vi "Change password GUI.vi"(6 "User access cluster in":T1 {"Expire sec" format="%.2f"}, 8 "error in (no error)":errorcluster, 10 "New user?":bool, 11 "Filepath":path=path "C:/Documents and Settings/default/Desktop/New Folder/passwords.log") -> (0 "error out":errorcluster, 1 "Activity log out":T3 {"Epoch sec" format="%.2e"}, 2 "Cancelled?":bool, 4 "User access cluster out":T1 {"Expire sec" format="%.2f"})   [LabVIEW 2013]
doc: "This is a pop-up panel which lets the user to enter a new password or click cancel (if \"New user?\" = F). It is a modal GUI.\n\nIt uses a filepath to an encrypted password file. If there is a file read error a custom error code is returned (error not announced here). \n\nIf called with \"New user?\" = F the user must enter both old and new passwords, else the old password is filled automaticallly from the \"User access cluster in\". The prompt also changes depending on the state of the \"new user?\" input.\n\nWhen the user clicks OK, the code:\n1) checks that old password is valid for this user, if not, it is announced, and this vi returns.\n2) checks that the two new passwords are identical. If not, user is informed and the vi waits for another continue or cancel (if enabled).\n3) If the two new passwords are equal, they are checked for minimum length of \"Min password char\" (from access configuration cluster) characters. If not of sufficient length, user is informed, and this vi waits for continue or cancel.\n4) finally, if new passwords are equal and valid this vi writes the new password to file. Also, if the user was a new user, this field is set to false in the password file.\n\n If the user changes the pasword it is recorded in the activity log, which can be written to an activity log file by subsequent vis."
uses:
  User Access Type defs/Acitivity cluster array.ctl
  User Access Type defs/Acitivity cluster.ctl
  User Access Type defs/User access cluster.ctl
  User Access Type defs/Security level U8.ctl
panel:
  in  "New password 2":string caption="New password\n(repeat)"
  in  "New password":string
  out "State case":string
  in  "Old password":string
  in  "Boolean 2":bool
  in  "Boolean":bool
  out "prompt":string="Enter your old password and the new password (twice)"
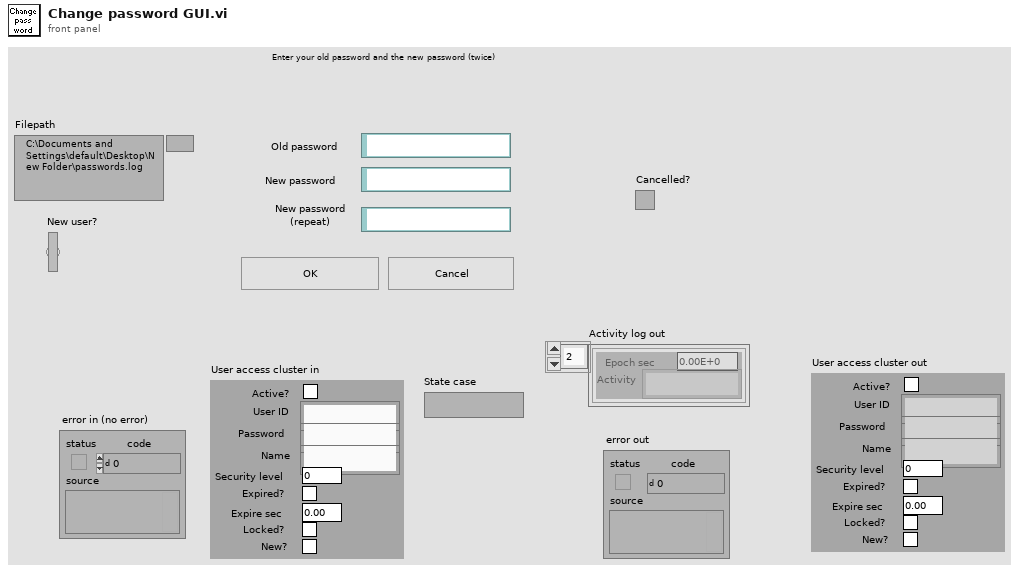
[diagram p1: front panel]
types:
  T1 = typedef "User access cluster.ctl" = cluster{"Active?":bool, "User ID":string, "Password":string, "Name":string, "Security level":T2, "Expired?":bool, "Expire sec":dbl, "Locked?":bool, "New?":bool}
  T2 = typedef "Security level U8.ctl" = u8
  T3 = typedef "Acitivity cluster array.ctl" = T4[]
  T4 = typedef "Acitivity cluster.ctl" = cluster{"Epoch sec":dbl, "Activity":string}
  T5 = typedef "All users access configuration cluster.ctl" = cluster{"Max ID attempts":i32, "Max password attempts":i32, "Expiration enabled":bool, "Expire days":i32, "User array":T6, "Min password char":i32}
  T6 = typedef "User access cluster array.ctl" = T1[]
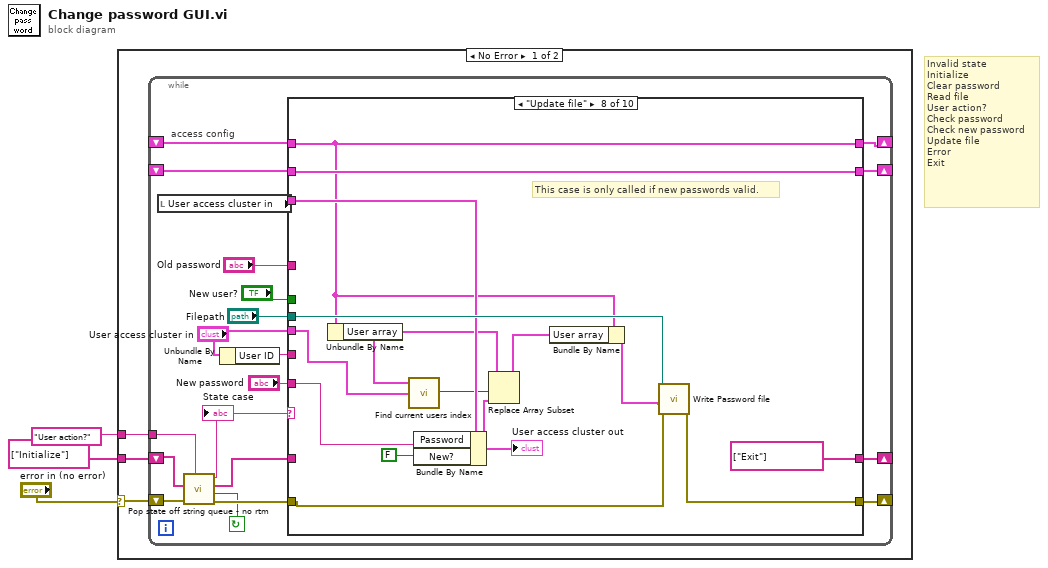
[diagram p0: block diagram]
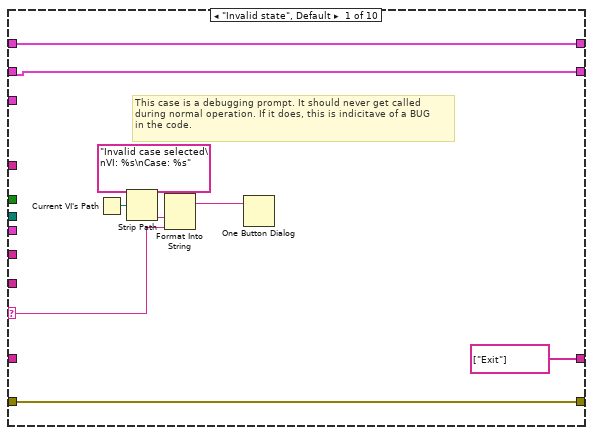
[diagram p2: hidden frame]
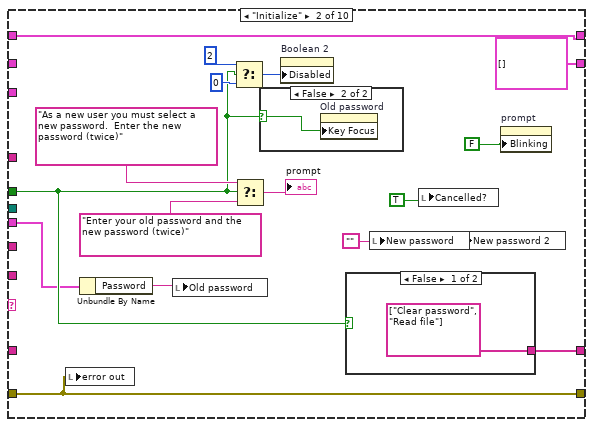
[diagram p3: hidden frame]
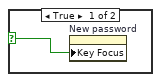
[diagram p4: hidden frame]
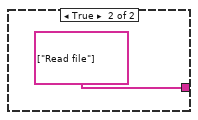
[diagram p5: hidden frame]
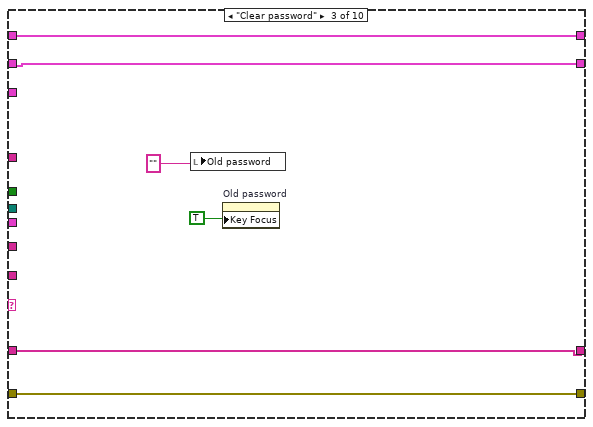
[diagram p6: hidden frame]
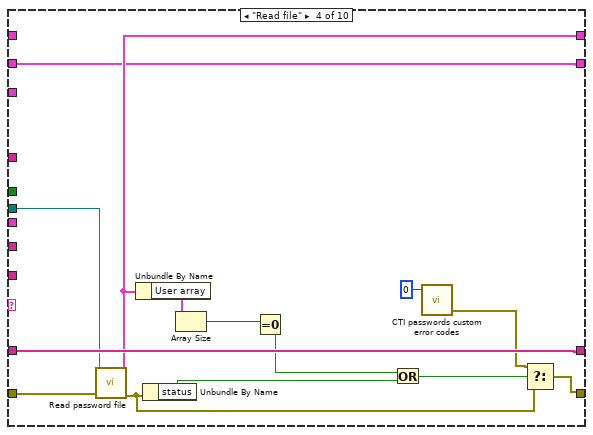
[diagram p7: hidden frame]
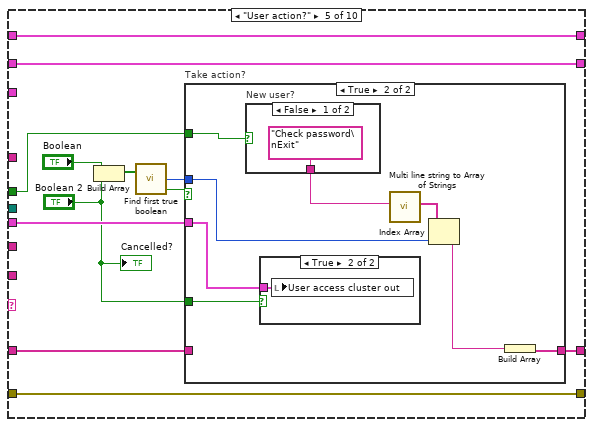
[diagram p8: hidden frame]
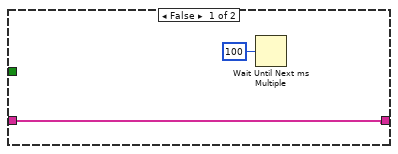
[diagram p9: hidden frame]
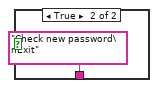
[diagram p11: hidden frame]
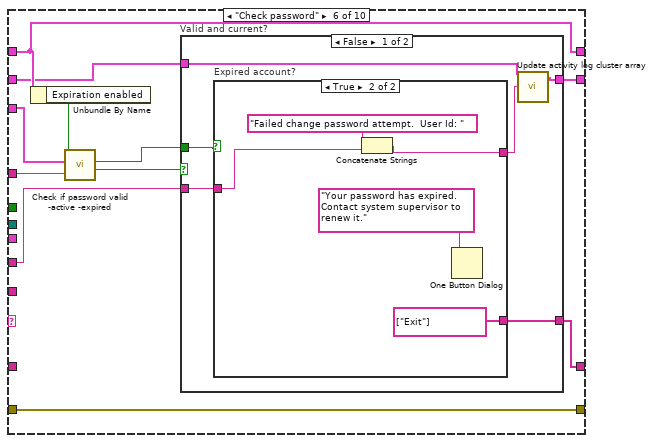
[diagram p12: hidden frame]
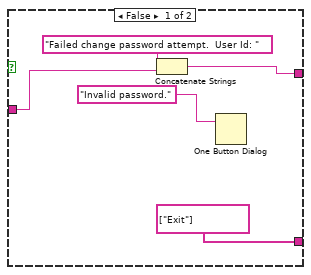
[diagram p13: hidden frame]
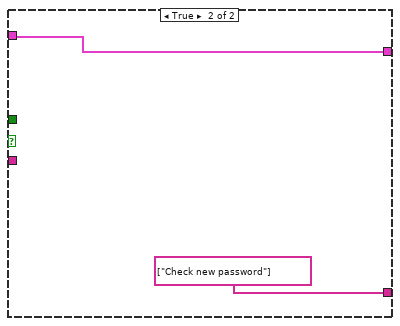
[diagram p14: hidden frame]
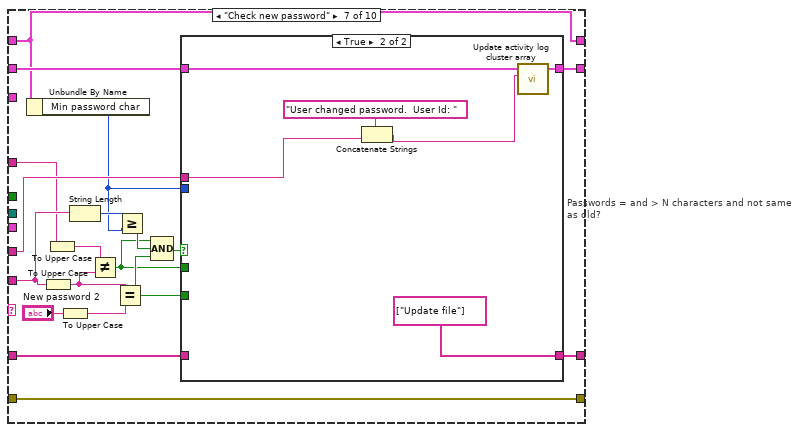
[diagram p15: hidden frame]
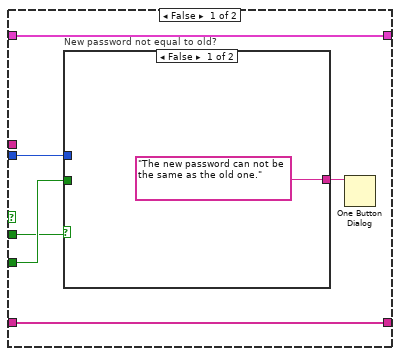
[diagram p16: hidden frame]
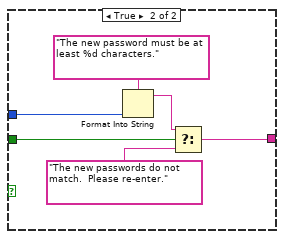
[diagram p17: hidden frame]
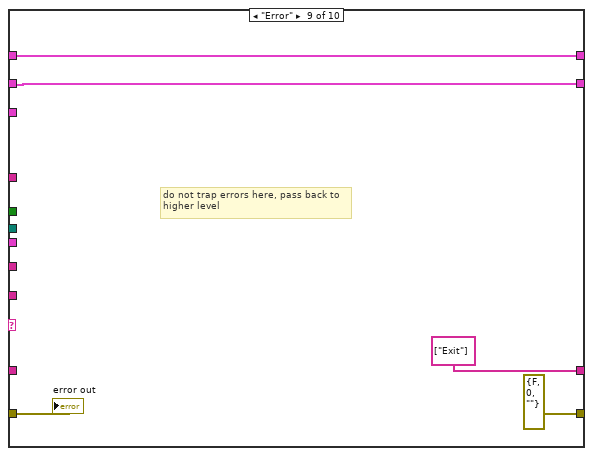
[diagram p18: hidden frame]
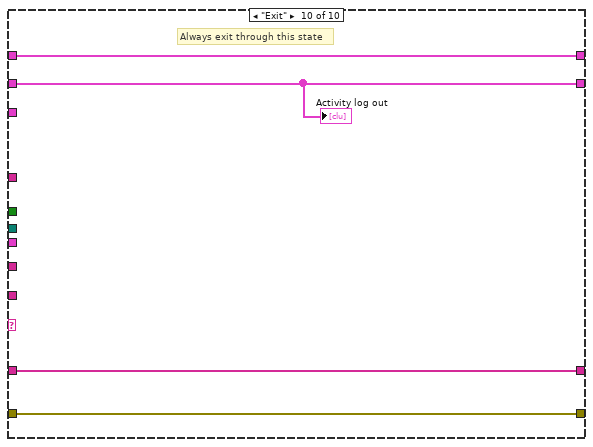
[diagram p19: hidden frame]
diagram:
  # "Invalid state\nInitialize\nClear password\nRead file\nUser action?\nCheck password\nCheck new password\nUpdate file\nError\nExit"
  n1 = case shown="No Error" "error in (no error)" {
    selector: "error in (no error)" -> [w6 _]
    tunnel: string[] ["Initialize"] ("State que out") -> [w5 _]
    tunnel: "User action?" ("Default state") -> [w4 _]
    frame No Error {
      n2 = while {
        tunnel: w4 -> [w18]
        shift-left: w5 -> [w22]
        shift-right: [w20] -> _
        shift-left: w6 -> [w26]
        shift-right: [w24] -> _
        shift-right: [w16] -> _
        shift-left: _ -> [w17]
        shift-right: [w15] -> _
        shift-left: _ -> [w14]
        stop <- w19 continue-if-true
        # "access config"
        n3 = local read "User access cluster in"() -> (w12:T1)
        n4 = call "Pop state off string queue - no rtm.vi"("Default state"=w18, "error in (no error)"=w26, "State que in"=w22) -> ("error out"=w25:errorcluster, "Not Exit?"=w19:bool, "State que out"=w21:string[], "State case"=w23:string)  [unwired: 5 out]
        "State case" <- w23
        n5 = Unbundle By Name("User access cluster in") -> ("User ID"=w10:string)
        n6 = case shown="\"Update file\"" w23 {
          selector: w23 -> [w30 _ _ _ _ _ _ _ _ _]
          tunnel: [w35 w51 w61 w68 w87 w111 w148 w180 errorcluster {"status"=FALSE, "code"=0, "source"=""} ("error out") w190] -> w24
          tunnel: w25 -> [w35 w51 w61 w74 w87 w111 w148 w179 w185 w190]
          tunnel: [string[] ["Exit"] ("State que out") w50 w57 w75 w86 w110 w147 string[] ["Exit"] ("State que out") string[] ["Exit"] ("State que out") w191] -> w20
          tunnel: w21 -> [_ _ w57 w75 w79 _ w142 _ _ w191]
          tunnel: [w28 w49 w59 w72 w84 w104 w143 w176 w183 w189] -> w16
          tunnel: w17 -> [w28 w49 w59 _ w84 w104 w143 w176 w183 w189]
          tunnel: w14 -> [w27 _ w58 w62 w85 w102 w145 w182 w184 w188]
          tunnel: [w27 T3 [] ("Activity log out") w58 w62 w85 w101 w144 w182 w184 w188] -> w15
          tunnel: "Filepath" -> [_ _ _ w73 _ _ _ w178 _ _]
          tunnel: w10 -> [_ _ _ _ _ w109 w146 _ _ _]
          tunnel: w12 -> [_ _ _ _ _ w107 _ w177 _ _]
          tunnel: "Old password" -> [_ _ _ _ _ w108 w133 _ _ _]
          tunnel: "New user?" -> [_ w41 _ _ w78 _ _ _ _ _]
          tunnel: "New password" -> [_ _ _ _ _ _ w139 w172 _ _]
          tunnel: "User access cluster in" -> [_ w40 _ _ w77 _ _ w170 _ _]
          frame "Invalid state", Default {
            # "This case is a debugging prompt. It should never get called\nduring normal operation. If it does, this is indicitave of a BUG\nin the code."
            n7 = Current VI's Path() -> (path=w32:path)
            n8 = Strip Path(path=w32) -> (name=w31:string)  [unwired: 1 out]
            n9 = Format Into String(format string="Invalid case selected\nVI: %s\nCase: %s" ("message"), w31, w30) -> (resulting string=w33:string)  [unwired: 2 in, 1 out]
            n10 = One Button Dialog(message=w33) -> ()  [unwired: 2 out]
          }
          frame "Initialize" {
            w38 = ""
            n11 = local write "error out"(w51) -> ()
            n12 = Unbundle By Name(w40) -> ("Password"=w39:string)
            n13 = local write "Old password"(w39) -> ()
            n14 = Select(t=u8 2 ("Disabled"), s=w41, f=u8 0 ("Disabled")) -> (s? t:f=w44:u8)
            n15 = Select(t="As a new user you must select a new password.  Enter the new password (twice)" ("prompt"), s=w41, f="Enter your old password and the new password (twice)" ("prompt")) -> (s? t:f=→"prompt":string)
            n16 = case shown="False" w41 {
              selector: w41 -> [w52 w53]
              frame True {
                n17 = property on="New password" class="Str"("Key Focus"=w52) -> ()  [unwired: 2 in, 2 out]
              }
              frame False {
                n18 = property on="Old password" class="Str"("Key Focus"=w53) -> ()  [unwired: 2 in, 2 out]
              }
            }
            n19 = property on="Boolean 2" class="Bool"("Disabled"=w44) -> ()  [unwired: 2 in, 2 out]
            n20 = case shown="False" w41 {
              tunnel: [string[] ["Clear password", "Read file"] ("State que out") string[] ["Read file"] ("State que out")] -> w50
              frame False {
              }
              frame True {
              }
            }
            n21 = local write "New password"(w38) -> ()
            n22 = local write "Cancelled?"(TRUE ("Valid password?")) -> ()
            n23 = local write "New password 2"(w38) -> ()
            n24 = property on="prompt" class="Str"("Blinking"=FALSE) -> ()  [unwired: 2 in, 2 out]
          }
          frame "Clear password" {
            n25 = local write "Old password"("" ("Password")) -> ()
            n26 = property on="Old password" class="Str"("Key Focus"=TRUE) -> ()  [unwired: 2 in, 2 out]
          }
          frame "Read file" {
            n27 = call "Read password file.vi"("error in (no error)"=w74, "file path"=w73) -> ("error out"=w69:errorcluster, "Access Configuration"=w72:T5)  [unwired: 8 out]
            n28 = Unbundle By Name(w72) -> ("User array"=w71:T6)
            n29 = Unbundle By Name(w69) -> ("status"=w66:bool)
            n30 = Array Size(array=w71) -> (size(s)=w70:i32)
            n31 = Equal To 0?(x=w70) -> (x = 0?=w67:bool)
            n32 = Or(x=w67, y=w66) -> (x .or. y?=w65:bool)
            n33 = call "CTI passwords custom error codes.vi"("error index"=0) -> ("error out"=w64:errorcluster)  [unwired: 1 in, 3 out]
            n34 = Select(t=w64, s=w65, f=w69) -> (s? t:f=w68:errorcluster)
          }
          frame "User action?" {
            n35 = Build Array("Boolean", "Boolean 2") -> (w82:bool[])
            n36 = call "Find first true boolean.vi"("Boolean Array IN"=w82) -> ("Index of first (T)"=w80:i32, "True found?"=w81:bool)  [unwired: 2 out]
            n37 = case "Take action?" shown="True" w81 {
              tunnel: [w89 w95] -> w86
              tunnel: w80 -> [_ w92]
              tunnel: w79 -> [w89 _]
              tunnel: w78 -> [_ w93]
              tunnel: w77 -> [_ w90]
              tunnel: "Boolean 2" -> [_ w91]
              frame False {
                n38 = Wait Until Next ms Multiple(millisecond multiple=u32 100) -> ()  [unwired: 1 out]
              }
              frame True {
                n39 = case "New user?" shown="False" w93 {
                  tunnel: ["Check password\nExit" ("Multi Line String") "Check new password\nExit" ("Multi Line String")] -> w94
                  frame False {
                  }
                  frame True {
                  }
                }
                n40 = case shown="True" w91 {
                  tunnel: w90 -> [_ w98]
                  frame False {
                  }
                  frame True {
                    n41 = local write "User access cluster out"(w98) -> ()
                  }
                }
                n42 = call "Multi line string to Array of Strings.vi"("Multi Line String"=w94) -> ("Array of Strings"=w97:string[])  [unwired: 6 out]
                n43 = Index Array(array=w97, index=w92) -> (element=w96:string)
                n44 = Build Array(w96) -> (w95:string[])
              }
            }
            "Cancelled?" <- "Boolean 2"
          }
          frame "Check password" {
            n45 = Unbundle By Name(w104) -> ("Expiration enabled"=w103:bool)
            n46 = call "Check if password valid -active -expired.vi"("Password"=w108, "User access cluster"=w107, "Expiration enabled?"=w103) -> ("Valid & current?"=w106:bool, "Expired?"=w105:bool)  [unwired: 1 in, 6 out]
            n47 = case "Valid and current?" shown="False" w106 {
              tunnel: [w117 string[] ["Check new password"] ("State que out")] -> w110
              tunnel: w109 -> [w116 _]
              tunnel: w105 -> [w115 _]
              tunnel: w102 -> [w114 w128]
              tunnel: [w113 w128] -> w101
              frame False {
                n48 = case "Expired account?" shown="True" w115 {
                  tunnel: [string[] ["Exit"] ("State que out") string[] ["Exit"] ("State que out")] -> w117
                  tunnel: w116 -> [w121 w126]
                  tunnel: [w120 w123] -> w112
                  frame False {
                    n49 = Concatenate Strings("Failed change password attempt.  User Id: ", w121) -> (w120:string)
                    n50 = One Button Dialog(message="Invalid password.") -> ()  [unwired: 2 out]
                  }
                  frame True {
                    n51 = Concatenate Strings("Failed change password attempt.  User Id: ", w126) -> (w123:string)
                    n52 = One Button Dialog(message="Your password has expired.  Contact system supervisor to renew it.") -> ()  [unwired: 2 out]
                  }
                }
                n53 = call "Update activity log cluster array.vi"("Activity description"=w112, "Activity log in"=w114) -> ("Activity log out"=w113:T3)  [unwired: 3 out]
              }
              frame True {
              }
            }
          }
          frame "Check new password" {
            n54 = Unbundle By Name(w143) -> ("Min password char"=w135:i32)
            n55 = To Upper Case(1:w139) -> (0:w131:string)
            n56 = To Upper Case(1:w133) -> (0:w132:string)
            n57 = To Upper Case(1:"New password 2") -> (0:w134:string)
            n58 = String Length(string=w139) -> (length=w138:i32)
            n59 = Not Equal?(x=w132, y=w131) -> (x != y?=w130:bool)
            n60 = Equal?(x=w131, y=w134) -> (x = y?=w137:bool)
            n61 = Greater Or Equal?(x=w138, y=w135) -> (x >= y?=w141:bool)
            n62 = Compound Arithmetic op=AND(w130, w141, w137) -> (w136:bool)
            n63 = case "Passwords = and > N characters and not same as old?" shown="True" w136 {
              tunnel: [w153 string[] ["Update file"] ("State que out")] -> w147
              tunnel: w146 -> [_ w166]
              tunnel: w145 -> [w154 w165]
              tunnel: [w154 w164] -> w144
              tunnel: w142 -> [w153 _]
              tunnel: w137 -> [w152 _]
              tunnel: w135 -> [w151 _]
              tunnel: w130 -> [w149 _]
              frame False {
                n64 = case "New password not equal to old?" shown="False" w149 {
                  tunnel: w152 -> [_ w161]
                  tunnel: w151 -> [_ w160]
                  tunnel: ["The new password can not be the same as the old one." ("message") w157] -> w150
                  frame False {
                  }
                  frame True {
                    n65 = Format Into String(format string="The new password must be at least %d characters." ("message"), w160) -> (resulting string=w158:string)  [unwired: 2 in, 1 out]
                    n66 = Select(t=w158, s=w161, f="The new passwords do not match.  Please re-enter." ("message")) -> (s? t:f=w157:string)
                  }
                }
                n67 = One Button Dialog(message=w150) -> ()  [unwired: 2 out]
              }
              frame True {
                n68 = Concatenate Strings("User changed password.  User Id: ", w166) -> (w163:string)
                n69 = call "Update activity log cluster array.vi"("Activity description"=w163, "Activity log in"=w165) -> ("Activity log out"=w164:T3)  [unwired: 3 out]
              }
            }
          }
          frame "Update file" {
            # "This case is only called if new passwords valid."
            n70 = Unbundle By Name(w176) -> ("User array"=w171:T6)
            n71 = call "Find current users index.vi"("User access cluster"=w170, "User array"=w171) -> ("index"=w169:i32)  [unwired: 3 out]
            n72 = Bundle By Name(cluster=w177, "Password"=w172, "New?"=FALSE) -> (w174:T1)
            "User access cluster out" <- w174
            n73 = Replace Array Subset(array=w171, new element=w174, index=w169) -> (w175:T6)
            n74 = Bundle By Name(cluster=w176, "User array"=w175) -> (w173:T5)
            n75 = call "Write Password file.vi"("error in (no error)"=w179, "Access Configuration"=w173, "Path"=w178) -> ("error out"=w180:errorcluster)  [unwired: 8 out]
          }
          frame "Error" {
            # "do not trap errors here, pass back to\nhigher level"
            "error out" <- w185
          }
          frame "Exit" {
            # "Always exit through this state"
            "Activity log out" <- w188
          }
        }
      }
    }
    frame Error {
    }
  }
